vi "Get package_template_enum.vi"(8 "error in (no error)":errorcluster, 11 "gRPCid":T1) -> (0 "error out":errorcluster, 2 "package_template_enum":T2, 3 "gRPCid out":T1)   [LabVIEW 2024, in "Service Template.lvlib"]
uses:
  Service Template.lvlib
  package_templatemessage.ctl
  gRPC lv Support/grpc-lvsupport/grpcId.ctl
  2ed25e12-861d-4677-8ead-ace2906b2041.vi
  gRPC lv Support/grpc-lvsupport/TranslateGrpcError.vi
  <vilib>/Utility/error.llb/Error Cluster From Error Code.vi
  gRPC lv Support/grpc-lvsupport/grpc-lvsupport.lvlib
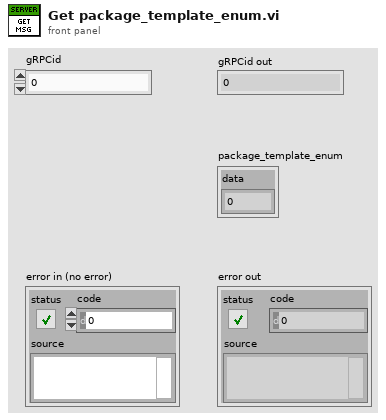
[diagram p1: front panel]
types:
  T1 = typedef "grpc-lvsupport.lvlib/grpcId.ctl" = u64
  T2 = typedef "Service Template.lvlib/package_templatemessage.ctl" = cluster{"data":sgl}
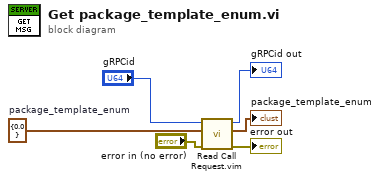
[diagram p0: block diagram]
diagram:
  w2 = T2 {"data"=0.0}  # package_template_enum
  n1 = call "Read Call Request.vim"("error in"="error in (no error)", "Request Type"=w2, "gRPCid in"="gRPCid") -> ("error out"=→"error out":errorcluster, "Request Data"=→"package_template_enum":T2, "gRPCid out"=→"gRPCid out":T1)  [unwired: 6 in]
